vi "Get Paths from Ref.vi"(8 "error in":errorcluster, 10 "Element to show log for":string, 11 "VI in":refnum<vi>) -> (0 "error out":errorcluster, 1 "/path":string, 2 "Working Directory":path, 3 "VI out":refnum<vi>)   [LabVIEW 2018, in "TortoiseGit Show Log.lvlib"]
doc: "Get the '/path' value for the VI based on whether the user asked to see the file/folder/class/library/repo log."
uses:
  TortoiseGit Show Log.lvlib
  <vilib>/Utility/error.llb/Error Cluster From Error Code.vi
  <vilib>/ErrorRing/Error Ring.xnode
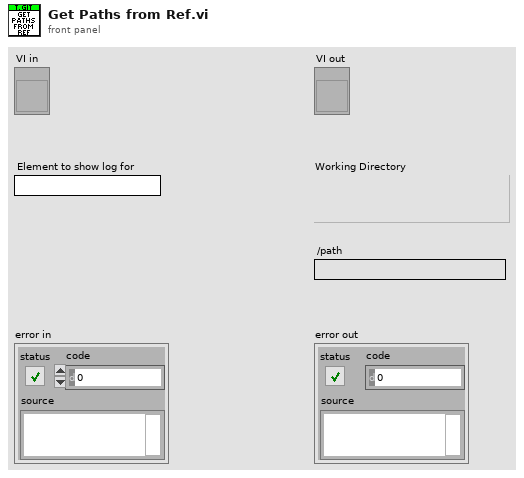
[diagram p1: front panel]
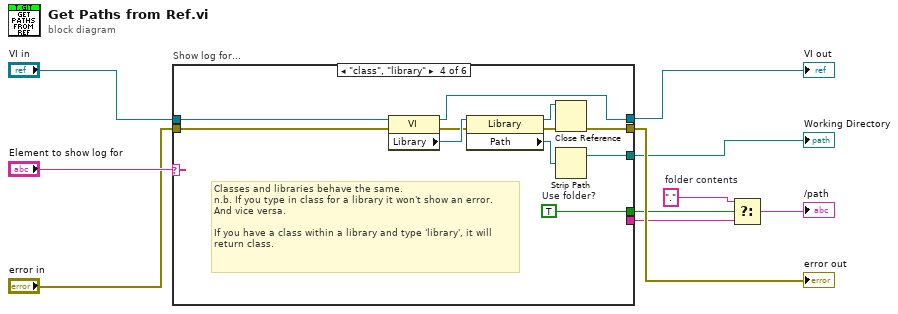
[diagram p0: block diagram]
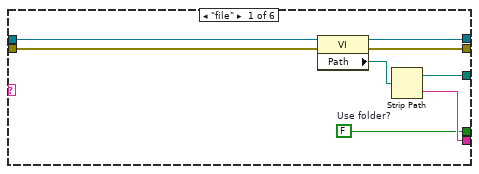
[diagram p2: hidden frame]
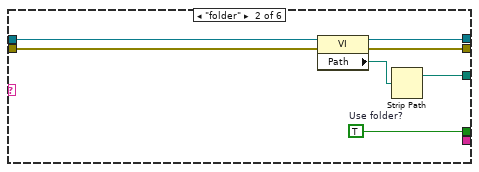
[diagram p3: hidden frame]
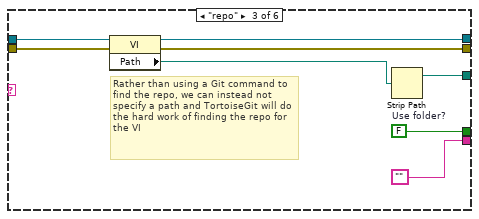
[diagram p4: hidden frame]
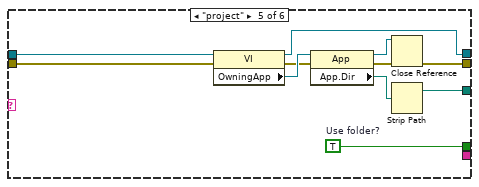
[diagram p5: hidden frame]
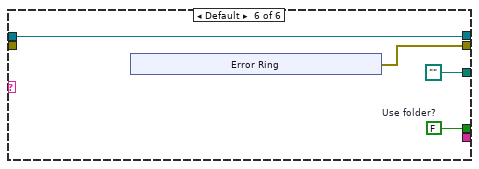
[diagram p6: hidden frame]
diagram:
  w8 = "."  # folder contents
  n1 = case "Show log for..." shown="\"class\", \"library\"" "Element to show log for" {
    tunnel: "VI in" -> [w18 w25 w29 w44 w55 w58]
    tunnel: [w16 _ "" _ _ _] -> w1
    tunnel: [w15 w23 w32 w35 w45 w57] -> w7
    tunnel: [w14 w22 w26 w36 w46 path ""] -> w9
    tunnel: [w13 w21 w28 w38 w49 w58] -> w4
    tunnel: "error in" -> [w12 w20 w33 w42 w53 _]
    tunnel: [w11 w19 w30 w41 w52 w59] -> w10
    frame "file" {
      w15 = FALSE  # Use folder?
      n2 = property class="VI"(reference=w18, error in=w12) -> (reference out=w13:refnum<vi>, error out=w11:errorcluster, "Path"=w17:path)
      n3 = Strip Path(path=w17) -> (stripped path=w14:path, name=w16:string)
    }
    frame "folder" {
      w23 = TRUE  # Use folder?
      n4 = property class="VI"(reference=w25, error in=w20) -> (reference out=w21:refnum<vi>, error out=w19:errorcluster, "Path"=w24:path)
      n5 = Strip Path(path=w24) -> (stripped path=w22:path)  [unwired: 1 out]
    }
    frame "repo" {
      w32 = FALSE  # Use folder?
      # "Rather than using a Git command to find the repo, we can instead not specify a path and TortoiseGit will do the hard work of finding the repo for the VI"
      n6 = property class="VI"(reference=w29, error in=w33) -> (reference out=w28:refnum<vi>, error out=w30:errorcluster, "Path"=w27:path)
      n7 = Strip Path(path=w27) -> (stripped path=w26:path)  [unwired: 1 out]
    }
    frame "class", "library" {
      w35 = TRUE  # Use folder?
      # "Classes and libraries behave the same.\nn.b. If you type in class for a library it won't show an error.\nAnd vice versa. \n\nIf you have a class within a library and type 'library', it will\nreturn class."
      n8 = property class="VI"(reference=w44, error in=w42) -> (reference out=w38:refnum<vi>, error out=w39:errorcluster, "Library"=w43:refnum<vi>)
      n9 = property class="Library"(reference=w43, error in=w39) -> (reference out=w40:refnum<vi>, error out=w37:errorcluster, "Path"=w34:path)
      n10 = Close Reference(reference=w40, error in (no error)=w37) -> (error out=w41:errorcluster)
      n11 = Strip Path(path=w34) -> (stripped path=w36:path)  [unwired: 1 out]
    }
    frame "project" {
      w45 = TRUE  # Use folder?
      n12 = property class="VI"(reference=w55, error in=w53) -> (reference out=w49:refnum<vi>, error out=w50:errorcluster, "OwningApp"=w54:refnum<vi>)
      n13 = property class="App"(reference=w54, error in=w50) -> (reference out=w51:refnum<vi>, error out=w48:errorcluster, "App.Dir"=w47:path)
      n14 = Close Reference(reference=w51, error in (no error)=w48) -> (error out=w52:errorcluster)
      n15 = Strip Path(path=w47) -> (stripped path=w46:path)  [unwired: 1 out]
    }
    frame Default {
      w57 = FALSE  # Use folder?
      n16 = xnode "Error Ring"() -> ("error out"=w59:errorcluster)
    }
  }
  "error out" <- w10
  "Working Directory" <- w9
  "VI out" <- w4
  n17 = Select(t=w8, s=w7, f=w1) -> (s? t:f=→"/path":string)
